vi "Create Bool Command Parameter.vi"(10 "Command Data":T1={"Address Areas"=131, "Data Block #"=0, "Start Address (bytes)"=104, "Write Data Float"=0.0, "Bit #"=0, "Write Data Boolean"=FALSE} {"Address Areas" items=["I/O (P)"=128, "Input (I)"=129, "Output (Q)"=130, "Bit Memory (M)"=131, "Data (DB)"=132, "Instance Data (DI)"=133, "Local Data (L)"=134, "Predecessor Local Data (VL)"=135]}, 11 "Cmd U16":u16 format="%x") -> (1 "Data Block #":u16, 2 "Start Address (bytes)":u32, 3 "Address Areas":u8, 5 "Cmd U16 out":u16 format="%x")   [LabVIEW 2018]
uses:
  CmdData.ctl
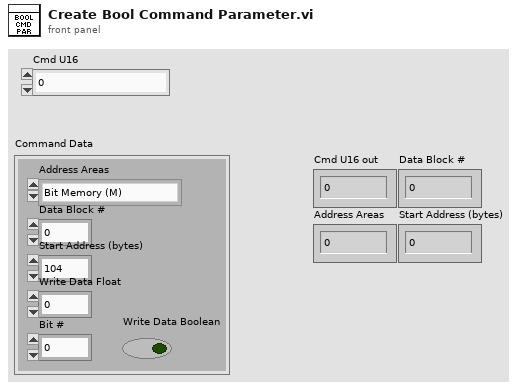
[diagram p1: front panel]
types:
  T1 = typedef "CmdData.ctl" = cluster{"Address Areas":u8, "Data Block #":u16, "Start Address (bytes)":u32, "Write Data Float":sgl, "Bit #":u16, "Write Data Boolean":bool}
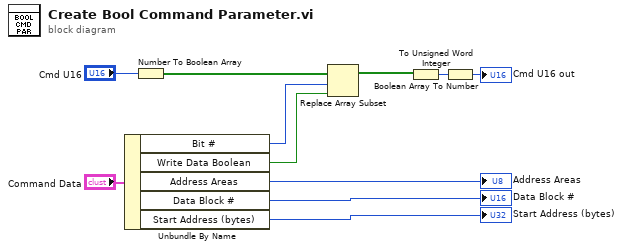
[diagram p0: block diagram]
diagram:
  n1 = Unbundle By Name("Command Data") -> ("Bit #"=w9:u16, "Write Data Boolean"=w8:bool, "Address Areas"=→"Address Areas":u8, "Data Block #"=→"Data Block #":u16, "Start Address (bytes)"=→"Start Address (bytes)":u32)
  n2 = Number To Boolean Array(number="Cmd U16") -> (Boolean array=w2:bool[])
  n3 = Replace Array Subset(array=w2, new element=w8, index=w9) -> (w1:bool[])
  n4 = Boolean Array To Number(Boolean array=w1) -> (number=w4:u32)
  n5 = To Unsigned Word Integer(number=w4) -> (unsigned 16bit integer=→"Cmd U16 out":u16)
